vi "Open HTML Report in Browser (Refnum).vi"(0 "report in":refnum<class "NI_report.lvclass">, 11 "error in (no error)":errorcluster) -> (4 "report out":refnum<class "NI_report.lvclass">, 6 "temporary HTML file created":path, 15 "error out":errorcluster)   [LabVIEW 2017, in "NI_ReportGenerationCore.lvlib"]
doc: "Displays an HTML report in the default Web browser. Wire data to the <B>report in</B> input to determine the polymorphic instance to use or manually select the instance. You cannot use this VI with standard reports."
uses:
  <vilib>/Utility/NIReport.llb/NI_ReportGenerationCore.lvlib
  <vilib>/Utility/NIReport.llb/NI_report.lvclass
  <vilib>/printing/ReportDocExtensions.llb/File_types_for_reports.ctl
  <vilib>/Platform/browser.llb/Open URL in Default Browser (string).vi
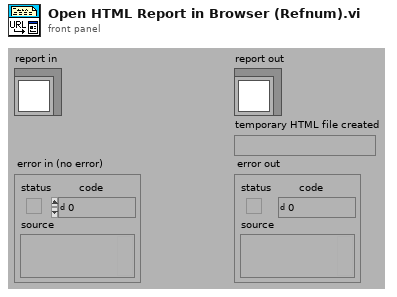
[diagram p1: front panel]
types:
  T1 = typedef "NI_ReportGenerationCore.lvlib/File_types_for_reports.ctl" = enum16{".jpg", ".png", ".html", ".gif"}
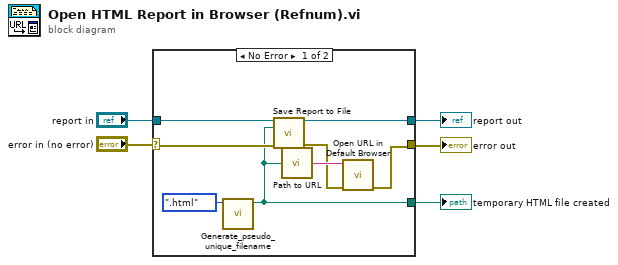
[diagram p0: block diagram]
diagram:
  n1 = case shown="No Error" "error in (no error)" {
    selector: "error in (no error)" -> [w12 w15]
    tunnel: [w8 w15] -> w4
    tunnel: "report in" -> [w11 w14]
    tunnel: [w7 _] -> w3
    tunnel: [w6 w14] -> w1
    frame No Error {
      n2 = call <vilib>:"Generate_pseudo_unique_filename.vi"("file type(.jpg)"=File_types_for_reports.".html") -> ("generated path"=w7:path)  [unwired: 8 in, 2 out]
      n3 = call-dynamic "Save Report to File.vi"("report in"=w11, "report file path"=w7, "error in (no error)"=w12) -> ("report out"=w6:refnum<class "NI_report.lvclass">, "error out"=w9:errorcluster)  [unwired: 11 in]
      n4 = call <vilib>:"Path to URL.vi"("path"=w7) -> ("url"=w10:string)
      n5 = call-poly <vilib>:"Open URL in Default Browser.vi"("error in (no error)"=w9, "URL"=w10) -> ("error out"=w8:errorcluster)  [unwired: 4 in, 1 out]
    }
    frame Error {
    }
  }
  "error out" <- w4
  "report out" <- w1
  "temporary HTML file created" <- w3
